vi "EnviraCom_Initialization.vi"(8 "error in (no error)":errorcluster, 11 "VISA Refnum in":refnum<visa-resource-name>) -> (0 "error out":errorcluster, 3 "VISA Refnum out":refnum<visa-resource-name>)   [LabVIEW 2023]
uses:
  <vilib>/Instr/_visa.llb/VISA Configure Serial Port (Instr).vi
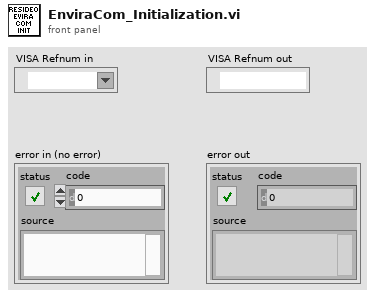
[diagram p1: front panel]
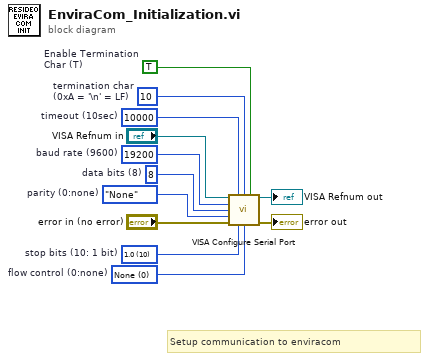
[diagram p0: block diagram]
diagram:
  w12 = TRUE  # Enable Termination Char (T)
  w11 = u32 10000  # timeout (10sec)
  w10 = u8 10  # termination char (0xA = '\n' = LF)
  w9 = u16 0 items=["None", "XON/XOFF", "RTS/CTS", "XON/XOFF & RTS/CTS", "DTR/DSR", "XON/XOFF & DTR/DSR"]  # flow control (0:none)
  w8 = u16 10 items=["1.0"=10, "1.5"=15, "2.0"=20]  # stop bits (10: 1 bit)
  w7 = enum16{"None", "Odd", "Even", "Mark", "Space"}."None"  # parity (0:none)
  w6 = u16 8  # data bits (8)
  w5 = u32 19200  # baud rate (9600)
  # "Setup communication to enviracom"
  n1 = call-poly "VISA Configure Serial Port"("VISA resource name"="VISA Refnum in", "timeout (10sec)"=w11, "termination char\n(0xA = '\\n' = LF)"=w10, "Enable Termination\nChar (T)"=w12, "baud rate (9600)"=w5, "data bits (8)"=w6, "parity (0:none)"=w7, "error in (no error)"="error in (no error)", "stop bits (10: 1 bit)"=w8, "flow control (0:none)"=w9) -> ("VISA resource name out"=→"VISA Refnum out":refnum<visa-resource-name>, "error out"=→"error out":errorcluster)  [unwired: 4 in]
